vi "SEQ Monitoring Global Variables.vi"() -> ()   [LabVIEW 2014]
uses:
  02_SEQ/TypeDefs/STEP.ctl
  02_SEQ/TypeDefs/LogicParsedExpression.ctl
  Mimico Display/TypeDefs/Mimic Data.ctl
  Mimico Display/TypeDefs/BG Image.ctl
  Mimico Display/TypeDefs/mObject.ctl
  02_SEQ/TypeDefs/Sequence.ctl
  02_SEQ/SeqLoop.lvlib
  Mimico Display/Mimico Display.lvlib
panel:
  in  "Sequence":T1
  in  "Current STEP":T2
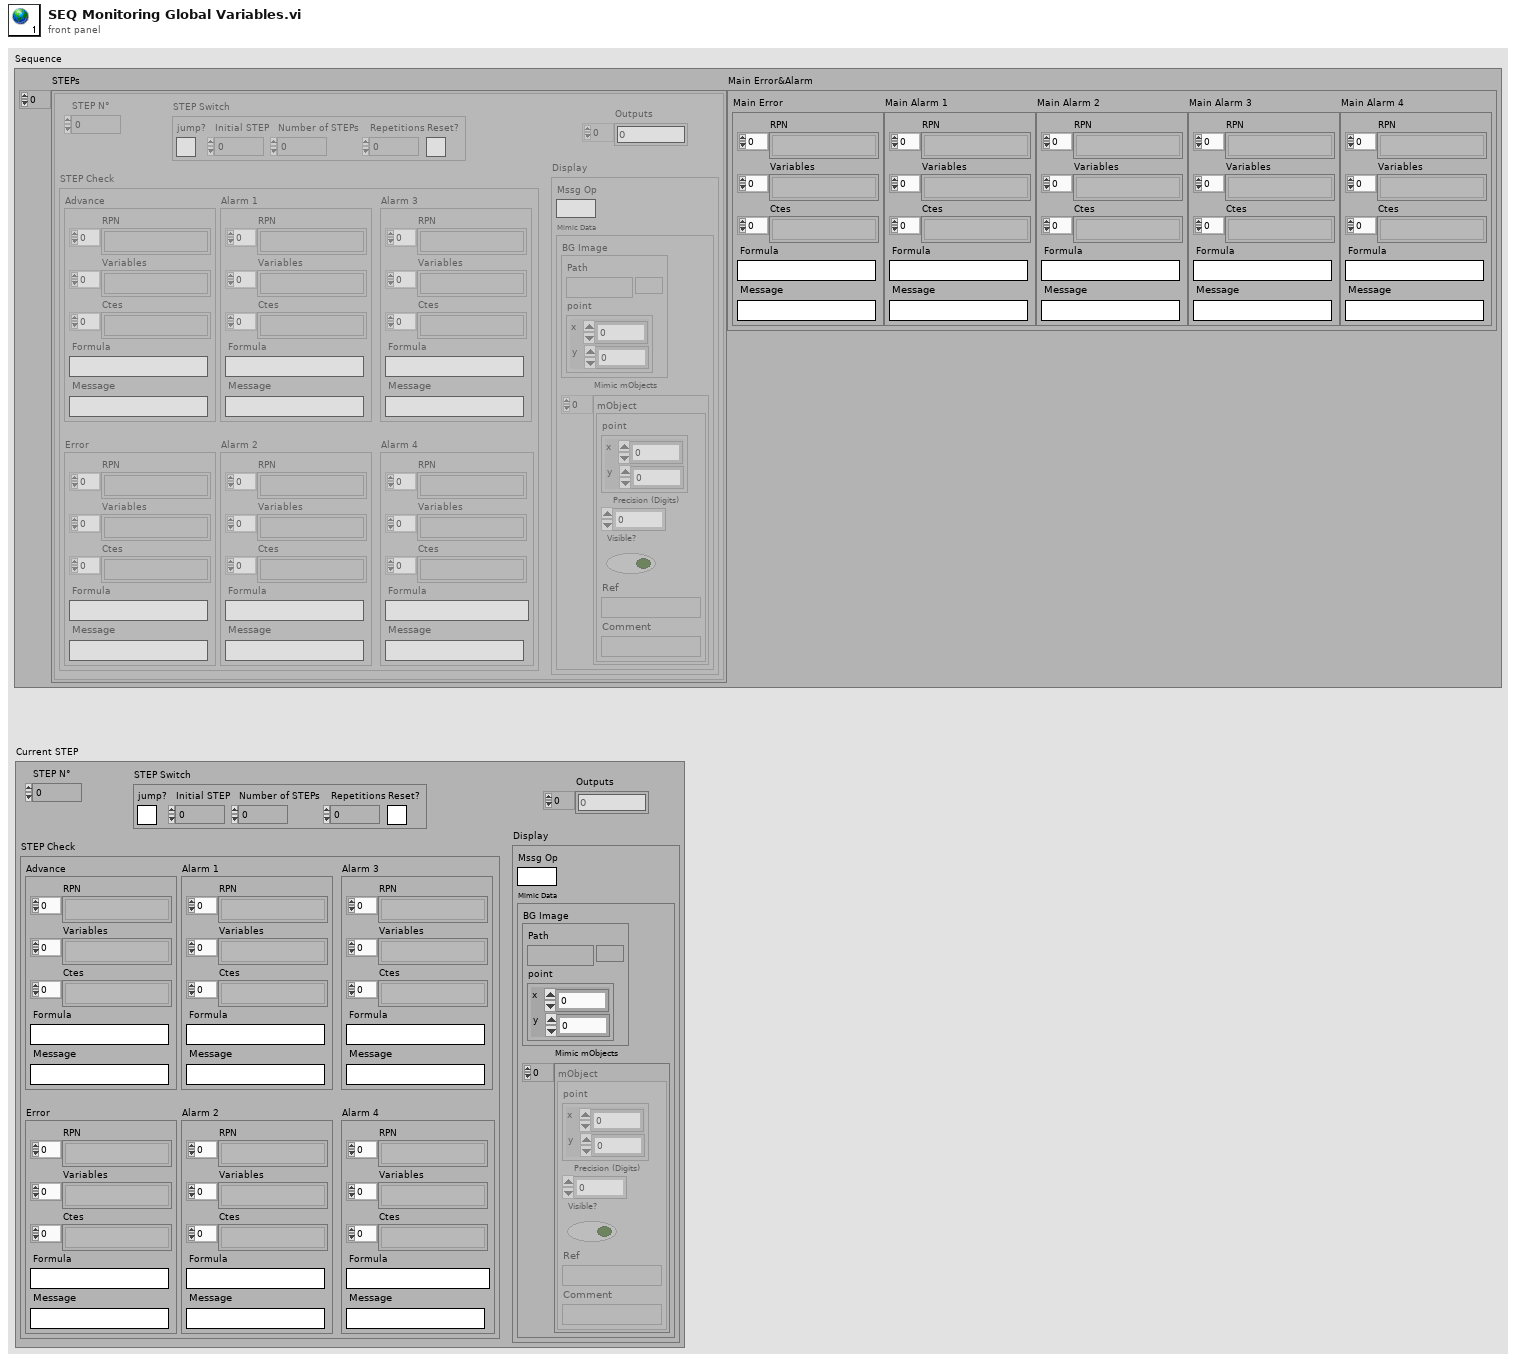
[diagram p1: front panel]
types:
  T1 = typedef "SeqLoop.lvlib/Sequence.ctl" = cluster{"STEPs":T2[], "Main Error&Alarm":cluster{"Main Error":T3, "Main Alarm 1":T3, "Main Alarm 2":T3, "Main Alarm 3":T3, "Main Alarm 4":T3}}
  T2 = typedef "SeqLoop.lvlib/STEP.ctl" = cluster{"STEP N°":u32, "STEP Switch":cluster{"jump?":bool, "Initial STEP":u32, "Number of STEPs":u32, "Repetitions":u32, "Reset?":bool}, "Outputs":i32[], "STEP Check":cluster{"Advance":T3, "Error ":T3, "Alarm 1":T3, "Alarm 2":T3, "Alarm 3":T3, "Alarm 4":T3}, "Display":cluster{"Mssg Op":string, "Mimic Data":T4}}
  T3 = typedef "SeqLoop.lvlib/LogicParsedExpression.ctl" = cluster{"RPN ":string[], "Variables":string[], "Ctes":string[], "Formula":string, "Message":string}
  T4 = typedef "SeqLoop.lvlib/Mimico Display.lvlib/Mimic Data.ctl" = cluster{"BG Image":T5, "Mimic mObjects":T6[]}
  T5 = typedef "SeqLoop.lvlib/Mimico Display.lvlib/BG Image.ctl" = cluster{"Path":path, "point":cluster{"x":i16, "y":i16}}
  T6 = typedef "SeqLoop.lvlib/Mimico Display.lvlib/mObject.ctl" = cluster{"point":cluster{"x":i16, "y":i16}, "Precision (Digits)":i32, "Visible?":bool, "Ref":string, "Comment":string}
diagram:
